vi "Parse Response Message.vi"(8 "error in":errorcluster, 11 "ThorlabsLabJack in":refnum<class "ThorlabsLabJack.lvclass">) -> (0 "error out":errorcluster, 3 "ThorlabsLabJack out":refnum<class "ThorlabsLabJack.lvclass">)   [LabVIEW 2018, in "ThorlabsLabJack.lvlib" / "ThorlabsLabJack.lvclass"]
doc: "This VI is in charge of querying and updating all the information about the Axis. This includes Position, Home Status, Moving Status, and whether there have been errors."
uses:
  ThorlabsLabJack.lvclass
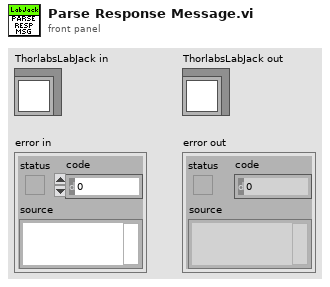
[diagram p1: front panel]
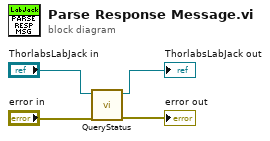
[diagram p0: block diagram]
diagram:
  n1 = call "QueryStatus.vi"("error in (no error)"="error in", "ThorlabsLabJack in"="ThorlabsLabJack in") -> ("error out"=→"error out":errorcluster, "ThorlabsLabJack out"=→"ThorlabsLabJack out":refnum<class "ThorlabsLabJack.lvclass">)  [unwired: 8 in]
